vi "oa_Make part of text in bold.vi"(8 "error in (no error)":errorcluster, 10 "Tips":string, 11 "Processed Tips":refnum<vi>) -> (0 "error out":errorcluster)   [LabVIEW 2017]
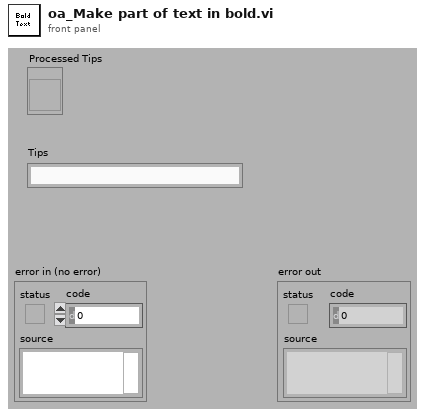
[diagram p1: front panel]
types:
  T1 = cluster{"offset past replacement":i32, "offset past replacement":i32}[]
  T2 = cluster{"offset past replacement":i32, "offset past replacement":i32}
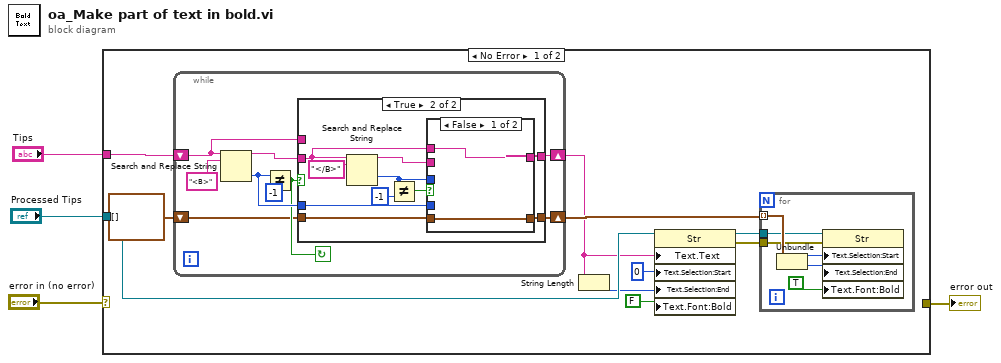
[diagram p0: block diagram]
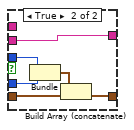
[diagram p3: hidden frame]
diagram:
  n1 = case shown="No Error" "error in (no error)" {
    selector: "error in (no error)" -> [_ w50]
    tunnel: "Tips" -> [w14 _]
    tunnel: [_ w50] -> w2
    tunnel: "Processed Tips" -> [w11 _]
    frame No Error {
      n2 = while {
        shift-right: [w24] -> w5
        shift-left: w14 -> [w25]
        shift-right: [w22] -> w13
        shift-left: T1 [] -> [w21]
        stop <- w23 continue-if-true
        n3 = Search and Replace String(input string=w25, search string="<B>" ("search string/char (-)")) -> (result string=w26:string, offset past replacement=w28:i32)  [unwired: 6 in, 2 out]
        n4 = Not Equal?(x=w28, y=-1) -> (x != y?=w23:bool)
        n5 = case shown="True" w23 {
          tunnel: [w31 w34] -> w24
          tunnel: w28 -> [_ w40]
          tunnel: w26 -> [_ w33]
          tunnel: w25 -> [w31 _]
          tunnel: [w30 w39] -> w22
          tunnel: w21 -> [w30 w38]
          frame False {
          }
          frame True {
            n6 = Search and Replace String(input string=w33, search string="</B>" ("search string/char (-)")) -> (result string=w35:string, offset past replacement=w36:i32)  [unwired: 6 in, 2 out]
            n7 = Not Equal?(x=w36, y=-1) -> (x != y?=w32:bool)
            n8 = case shown="False" w32 {
              tunnel: w40 -> [_ w49]
              tunnel: [w43 w47] -> w39
              tunnel: w38 -> [w43 w46]
              tunnel: w36 -> [_ w45]
              tunnel: w35 -> [_ w44]
              tunnel: [w42 w44] -> w34
              tunnel: w33 -> [w42 _]
              frame False {
              }
              frame True {
                n9 = Bundle("offset past replacement"=w49, "offset past replacement"=w45) -> (w48:T2)  [unwired: 1 in]
                n10 = Build Array (concatenate)(w48, w46) -> (w47:T1)
              }
            }
          }
        }
      }
      n11 = String Length(string=w5) -> (length=w9:i32)
      n12 = property class="Str"(reference=w11, "Text.Text"=w5, "Text.Selection:Start"=u32 0, "Text.Selection:End"=w9, "Text.Font:Bold"=FALSE) -> (reference out=w6:refnum<vi>, error out=w7:errorcluster)  [unwired: 1 in]
      n13 = for {
        tunnel: w13 -> [w20] mode=indexing
        tunnel: w7 -> [w18]
        tunnel: w6 -> [w19]
        n14 = Unbundle(w20) -> ("offset past replacement"=w15:i32, "offset past replacement"=w16:i32)
        n15 = property class="Str"(reference=w19, error in=w18, "Text.Selection:Start"=w15, "Text.Selection:End"=w16, "Text.Font:Bold"=TRUE) -> ()  [unwired: 2 out]
      }
    }
    frame Error {
    }
  }
  "error out" <- w2
